vi "Get Instruments.vi"(8 "Error In":errorcluster) -> (0 "Error Out":errorcluster, 2 "IInstruments":map{string, refnum<class "IInstrument.lvclass">}(c390))   [LabVIEW 2024, in "Instrument Manager.lvclass"]
uses:
  Instrument Manager.lvclass
  Interfaces/IInstrument/IInstrument.lvclass
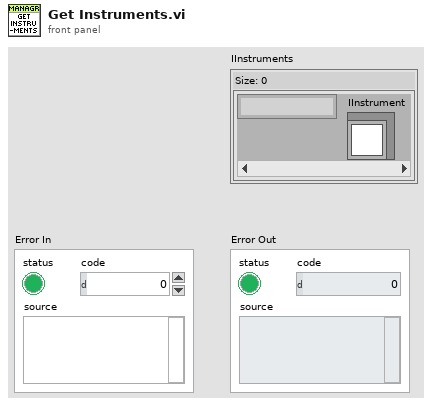
[diagram p1: front panel]
types:
  T1 = typedef "Instrument Manager.lvclass/ObjectAttributes.ctl" = cluster{"IInstruments":map{string, refnum<class "IInstrument.lvclass">}, "Instrument Configurations":map{string, refnum<class "Config from JSON.lvclass">}, "IVirtual Instruments":map{string, refnum<class "IVirtual Instrument.lvclass">}, "Virtual Instrument Configurations":map{string, refnum<class "Config from JSON.lvclass">}}
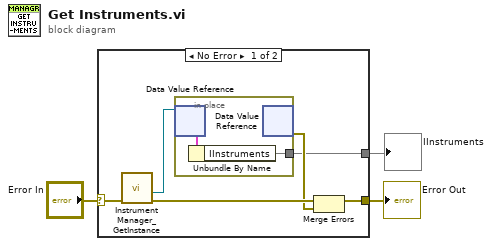
[diagram p0: block diagram]
diagram:
  n1 = case shown="No Error" "Error In" {
    selector: "Error In" -> [w9 w12]
    tunnel: [w7 w12] -> w2
    tunnel: [w5 _] -> w1
    frame No Error {
      n2 = call "Instrument Manager_GetInstance.vi"("Error In"=w9) -> ("Error Out"=w8:errorcluster, "DVRRefOut"=w4:refnum<data-value>)  [unwired: 6 in, 3 out]
      n3 = in-place {
        in-place-border: [w11] -> w5
        n4 = in-place-dvr #1(w4) -> (w10:T1)  [unwired: 1 out]
        n5 = Unbundle By Name(w10) -> ("IInstruments"=w11:map{string, refnum<class "IInstrument.lvclass">})
        n6 = in-place-dvr #1() -> (w6:errorcluster)  [unwired: 1 in, 1 out]
      }
      n7 = Merge Errors(w8, w6) -> (w7:errorcluster)
    }
    frame Error {
    }
  }
  "Error Out" <- w2
  "IInstruments" <- w1
